vi "Unflatten FIFO Config.vi"(7 "offset in":i32, 11 "Flattened Data in":u8[](array[numeric])) -> (3 "FIFO Config out":T1, 5 "offset out":i32)   [LabVIEW 2021, in "ChannelCommon.lvlib"]
uses:
  ChannelCommon.lvlib
  <vilib>/CIF Foundation/CIF Utilities/DataTypes/DataTypes_CIF_U.lvlib
  typedef/FIFO Config.ctl
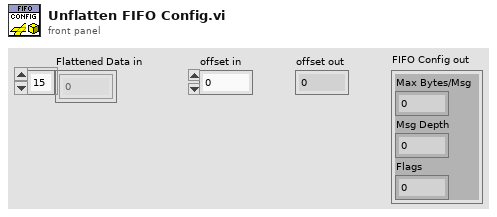
[diagram p1: front panel]
types:
  T1 = typedef "ChannelCommon.lvlib/FIFO Config.ctl" = cluster{"Max Bytes/Msg":u64, "Msg Depth":u64, "Flags":u64}
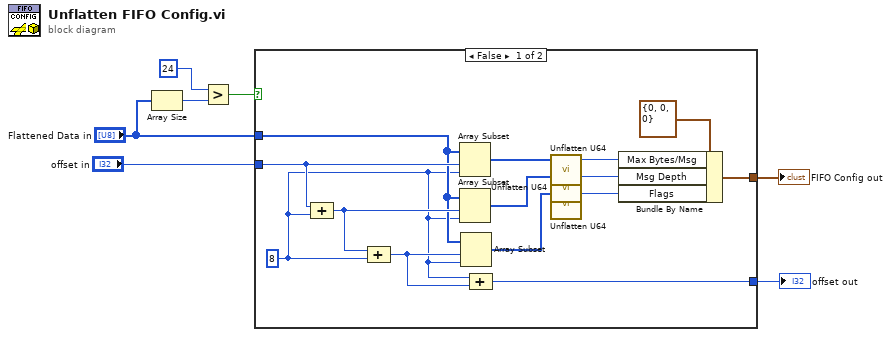
[diagram p0: block diagram]
diagram:
  n1 = Array Size(array="Flattened Data in") -> (size(s)=w3:i32)
  n2 = Greater?(x=24, y=w3) -> (0:w1:bool)
  n3 = case shown="False" w1 {
    tunnel: "offset in" -> [w20 _]
    tunnel: [w18 _] -> w6
    tunnel: [w12 _] -> w5
    tunnel: "Flattened Data in" -> [w10 _]
    frame False {
      w8 = 8 ("length")
      n4 = Compound Arithmetic op=ADD(w20, w8) -> (w14:i32)
      n5 = Compound Arithmetic op=ADD(w14, w8) -> (w13:i32)
      n6 = Array Subset(array=w10, index=w20, length=w8) -> (w21:u8[])
      n7 = Array Subset(array=w10, index=w14, length=w8) -> (w16:u8[])
      n8 = Array Subset(array=w10, index=w13, length=w8) -> (w11:u8[])
      n9 = Compound Arithmetic op=ADD(w8, w13) -> (w12:i32)
      n10 = call <vilib>:"Unflatten U64.vi"("Flat Data"=w21) -> ("U64"=w19:u64)  [unwired: 4 in]
      n11 = call <vilib>:"Unflatten U64.vi"("Flat Data"=w16) -> ("U64"=w15:u64)  [unwired: 4 in]
      n12 = call <vilib>:"Unflatten U64.vi"("Flat Data"=w11) -> ("U64"=w9:u64)  [unwired: 4 in]
      n13 = Bundle By Name(cluster=T1 {"Max Bytes/Msg"=0, "Msg Depth"=0, "Flags"=0} ("FIFO Config out 2"), "Max Bytes/Msg"=w19, "Msg Depth"=w15, "Flags"=w9) -> (w18:T1)
    }
    frame True {
    }
  }
  "FIFO Config out" <- w6
  "offset out" <- w5
